vi "Magnetometer - Convert 2's Complement Little Endian to I16_SubVI.vi"(10 "High Byte":u8, 11 "Low Byte":u8) -> (1 "Output I16":i16)   [LabVIEW 2021]
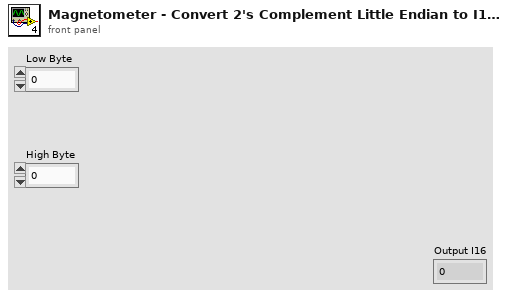
[diagram p1: front panel]
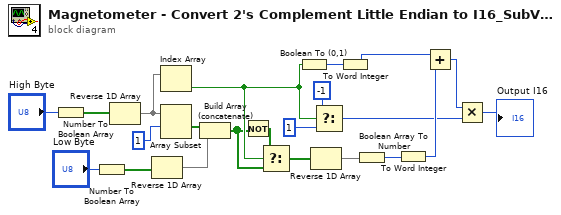
[diagram p0: block diagram]
diagram:
  n1 = Number To Boolean Array(number="High Byte") -> (Boolean array=w4:bool[])
  n2 = Number To Boolean Array(number="Low Byte") -> (Boolean array=w6:bool[])
  n3 = Reverse 1D Array(array=w4) -> (reversed array=w3:bool[])
  n4 = Reverse 1D Array(array=w6) -> (reversed array=w5:bool[])
  n5 = Index Array(array=w3) -> (element=w12:bool)  [unwired: 1 in]
  n6 = Array Subset(array=w3, index=1) -> (w22:bool[])  [unwired: 1 in]
  n7 = Build Array (concatenate)(w22, w5) -> (w10:bool[])
  n8 = Not(x=w10) -> (.not. x?=w11:bool[])
  n9 = Select(t=w11, s=w12, f=w10) -> (s? t:f=w8:bool[])
  n10 = Boolean To (0,1)(Boolean=w12) -> (0, 1=w14:i16)
  n11 = Reverse 1D Array(array=w8) -> (reversed array=w7:bool[])
  n12 = Select(t=i16 -1, s=w12, f=i16 1) -> (s? t:f=w2:i16)
  n13 = To Word Integer(number=w14) -> (16bit integer=w13:i16)
  n14 = Boolean Array To Number(Boolean array=w7) -> (number=w19:u32)
  n15 = To Word Integer(number=w19) -> (16bit integer=w9:i16)
  n16 = Add(x=w13, y=w9) -> (x+y=w1:i16)
  n17 = Multiply(x=w1, y=w2) -> (x*y=→"Output I16":i16)
